vi "SamsGrapher.vi"() -> ()   [LabVIEW 2016]
uses:
  inventory type def.ctl
  subscription type def.ctl
  Communication Global variables.vi
  <vilib>/addons/_JKI.lib/Serialization/JSON/JKI JSON Serialization.lvlib
panel:
  in  "Tab Control":enum32{"Controls", "Graph"}(tab)
  in  "Save Config":bool
  in  "refresh list":bool
  in  "Device selection":i32(listbox)
  in  "Selected parameters":i32[](listbox)
  in  "Available parameters":i32[](listbox)
  in  "Config Button":bool
  out "Data rate (hz)":dbl(knob) scale=0.0..200.0
  in  "Enable graphing":bool=TRUE
  out "Waveform chart":waveform(dbl)[](graph)=[{"t0"=timestamp(3553447770.6895175 s since 1904-01-01), "dt"=1.0, "Y"=[0.0]}, {"t0"=timestamp(3553447770.6895175 s since 1904-01-01), "dt"=1.0, "Y"=[nan]}, {"t0"=timestamp(3553447770.6895175 s since 1904-01-01), "dt"=1.0, "Y"=[nan]}, {"t0"=timestamp(3553447770.6895175 s since 1904-01-01), "dt"=1.0, "Y"=[nan]}, {"t0"=timestamp(3553447770.6895175 s since 1904-01-01), "dt"=1.0, "Y"=[nan]}, {"t0"=timestamp(3553447770.6895175 s since 1904-01-01), "dt"=1.0, "Y"=[nan]}, {"t0"=timestamp(3553447770.6895175 s since 1904-01-01), "dt"=1.0, "Y"=[nan]}, {"t0"=timestamp(3553447770.6895175 s since 1904-01-01), "dt"=1.0, "Y"=[nan]}, {"t0"=timestamp(3553447770.6895175 s since 1904-01-01), "dt"=1.0, "Y"=[nan]}, {"t0"=timestamp(3553447770.6895175 s since 1904-01-01), "dt"=1.0, "Y"=[nan]}, {"t0"=timestamp(3553447770.6895175 s since 1904-01-01), "dt"=1.0, "Y"=[nan]}, {"t0"=timestamp(3553447770.6895175 s since 1904-01-01), "dt"=1.0, "Y"=[nan]}, {"t0"=timestamp(3553447770.6895175 s since 1904-01-01), "dt"=1.0, "Y"=[nan]}, {"t0"=timestamp(3553447770.6895175 s since 1904-01-01), "dt"=1.0, "Y"=[nan]}, {"t0"=timestamp(3553447770.6895175 s since 1904-01-01), "dt"=1.0, "Y"=[nan]}, {"t0"=timestamp(3553447770.6895175 s since 1904-01-01), "dt"=1.0, "Y"=[nan]}]
  out "initialize error":errorcluster
  out "error out":errorcluster
  in  "stop":bool
  # "Parameter Selection"
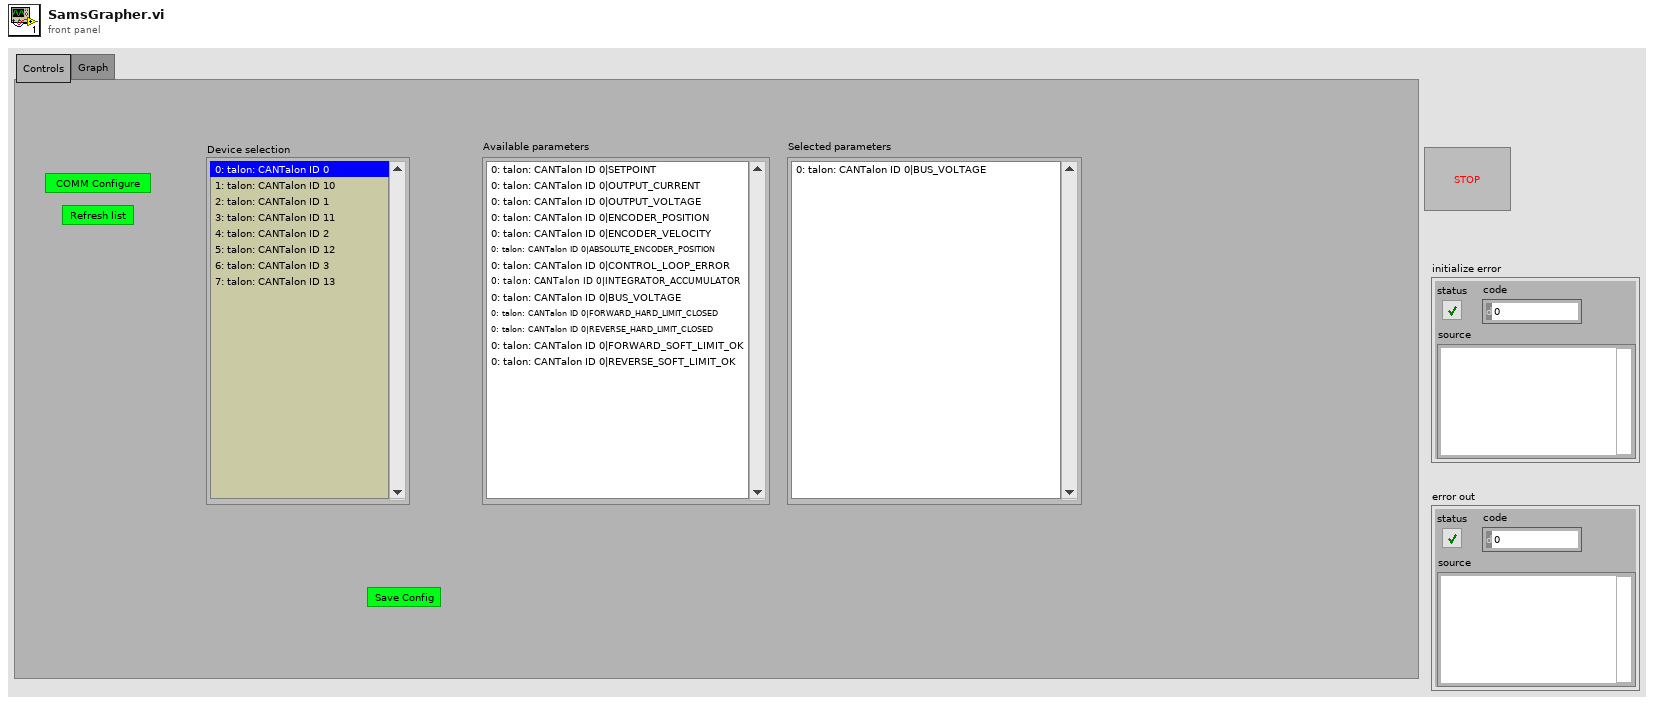
[diagram p1: front panel]
types:
  T1 = typedef "subscription type def.ctl" = cluster{"type":string, "subscription":cluster{"itemId":i32, "measurementId":string}[]}
  T2 = typedef "inventory type def.ctl" = cluster{"items":cluster{"id":u8, "type":string, "description":string}[], "measures":cluster{"deviceType":string, "deviceMeasures":cluster{"id":string, "description":string}[]}[], "type":string}
  T3 = cluster{"type":string, "timestamp":i64, "data":dbl[]}
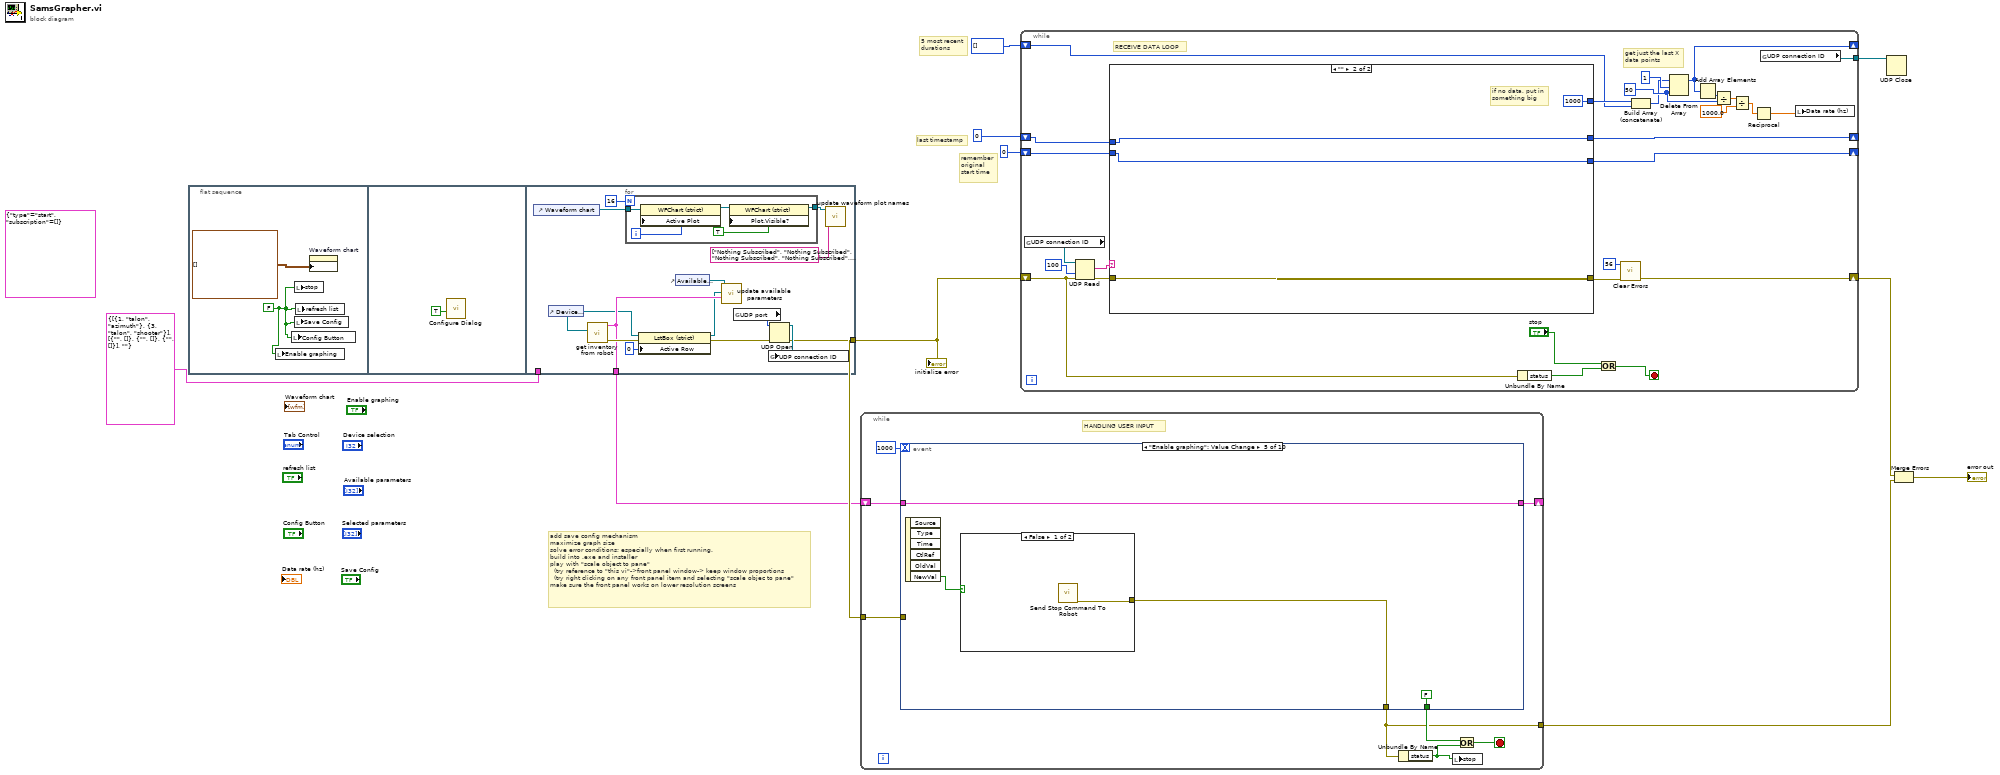
[diagram p0: block diagram]
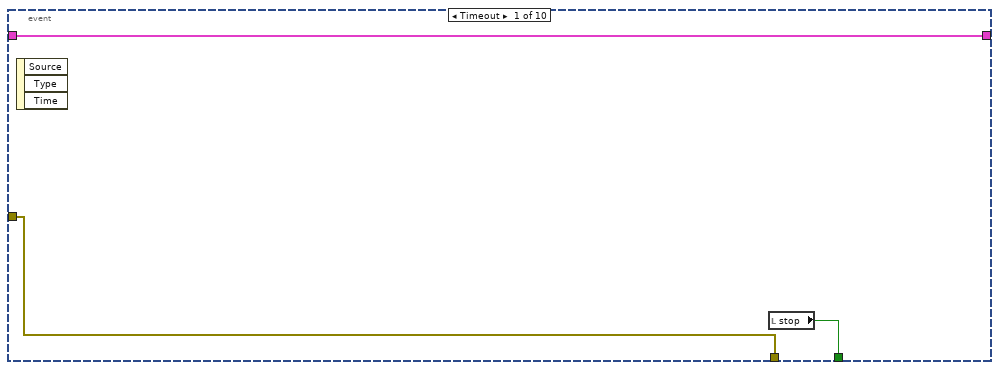
[diagram p2: hidden frame]
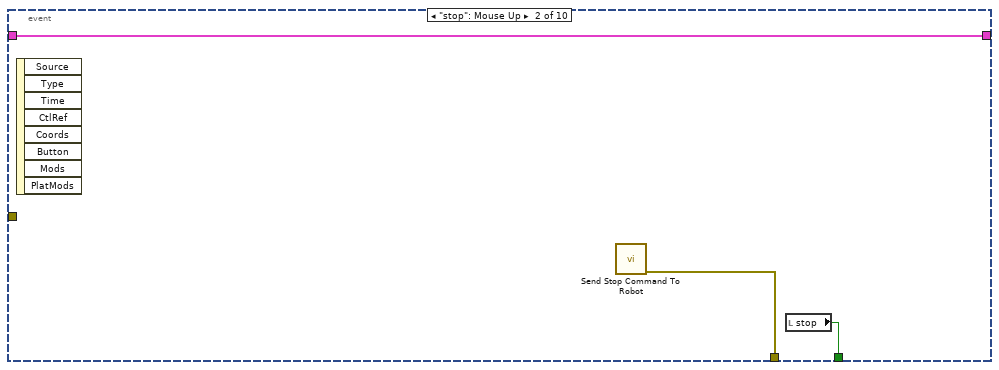
[diagram p3: hidden frame]
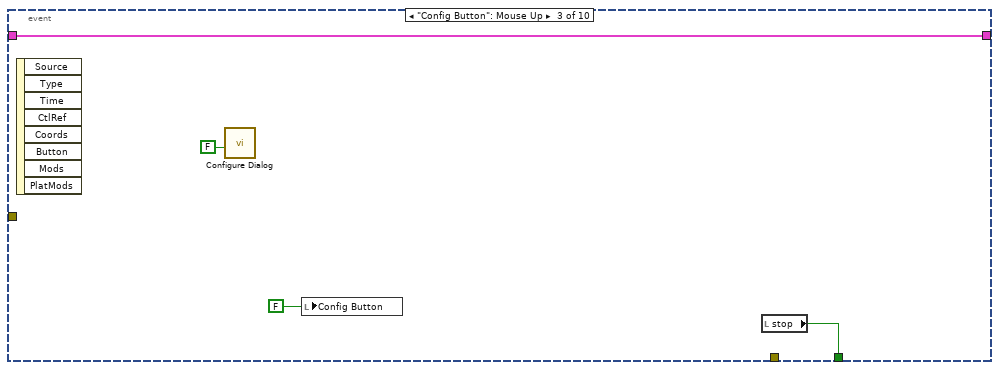
[diagram p4: hidden frame]
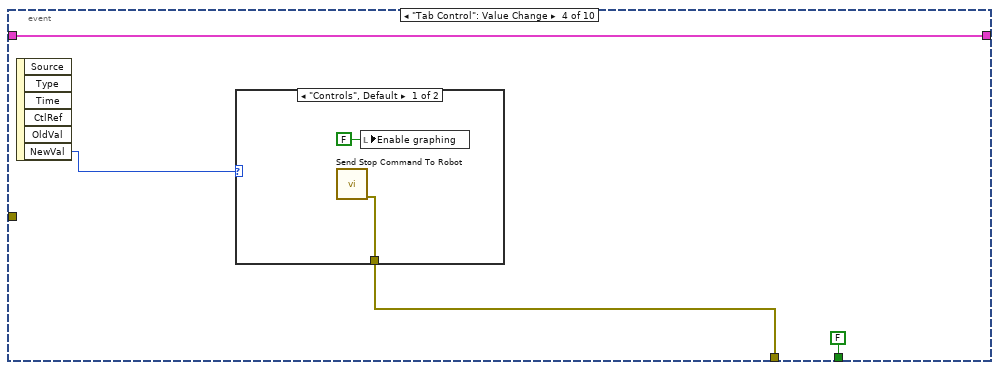
[diagram p5: hidden frame]
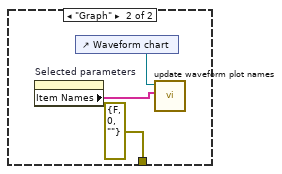
[diagram p6: hidden frame]
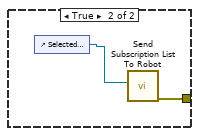
[diagram p7: hidden frame]
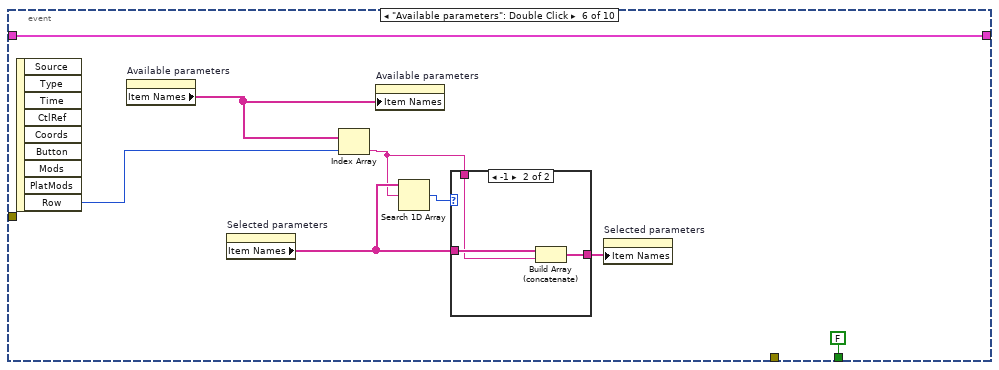
[diagram p8: hidden frame]
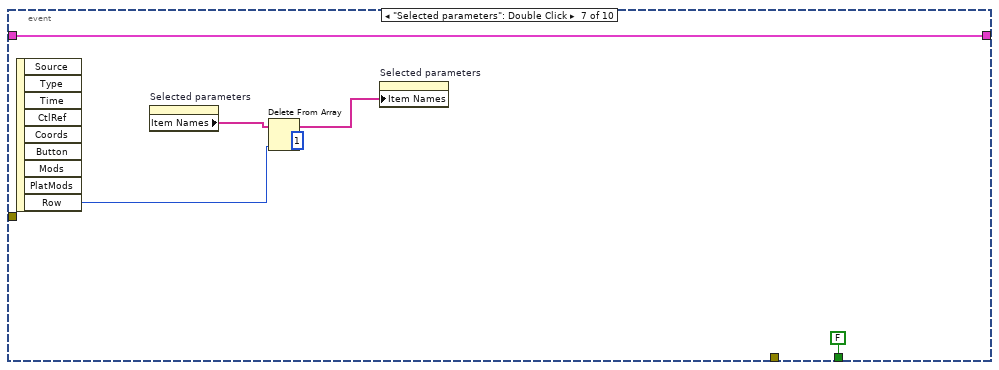
[diagram p10: hidden frame]
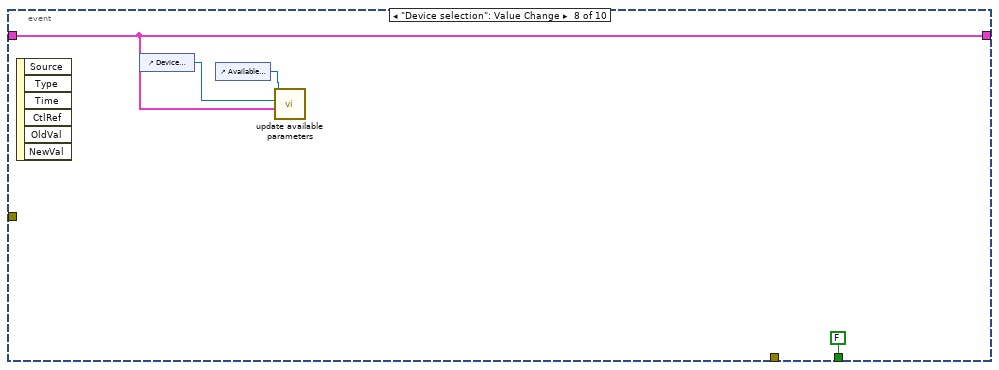
[diagram p11: hidden frame]
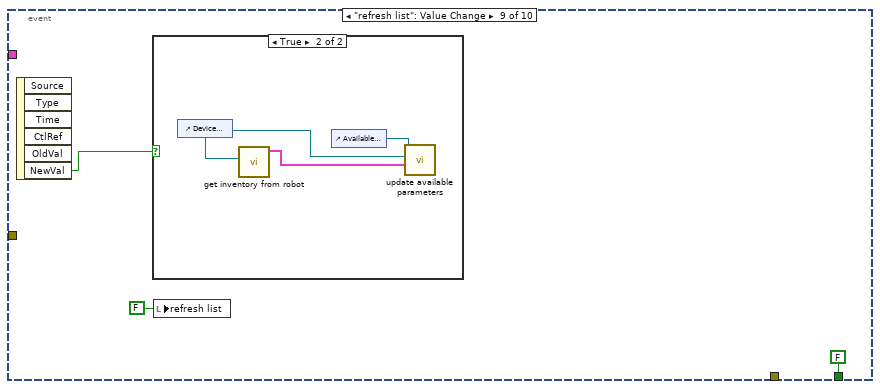
[diagram p12: hidden frame]
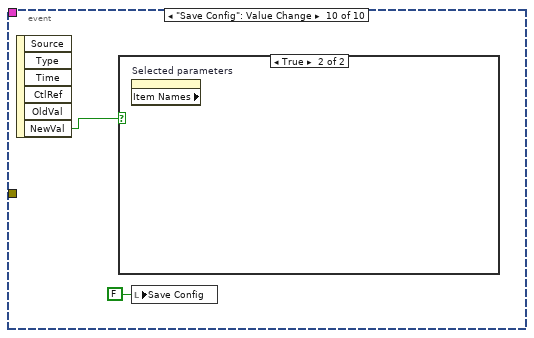
[diagram p14: hidden frame]
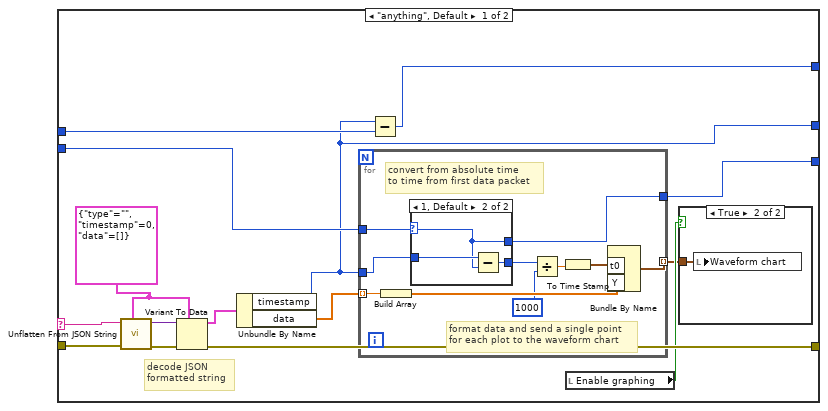
[diagram p16: hidden frame]
diagram:
  (unwired) T1 {"type"="start", "subscription"=[]}
  # "last timestamp"
  # "remember\noriginal\nstart time"
  # "5 most recent\ndurations"
  # "add save config mechanism\nmaximize graph size\nsolve error conditions; especially when first running.\nbuild into .exe and installer\nplay with \"scale object to pane\" \n  (try reference to \"this vi\"->front panel window-> keep window proportions\n  (try right clicking on any front panel item and selecting \"scale objec to pane\"\nmake sure the front panel works on lower resolution screens"
  n1 = flat-sequence {
    tunnel: [w25] -> w7
    tunnel: [w16] -> w6
    tunnel: T2 {"items"=[{"id"=1, "type"="talon", "description"="azimuth"}, {"id"=3, "type"="talon", "description"="shooter"}], "measures"=[{"deviceType"="", "deviceMeasures"=[]}, {"deviceType"="", "deviceMeasures"=[]}, {"deviceType"="", "deviceMeasures"=[]}], "type"=""} -> [_]
    frame #0 {
      w11 = FALSE ("Send")
      n2 = local write "Enable graphing"(w11) -> ()
      n3 = local write "Config Button"(w11) -> ()
      n4 = local write "Save Config"(w11) -> ()
      n5 = local write "stop"(w11) -> ()
      n6 = local write "refresh list"(w11) -> ()
      n7 = property on="Waveform chart" class="WFChart (strict)"("History Data"=waveform(dbl)[][] []) -> ()  [unwired: 2 in, 2 out]
    }
    frame #1 {
      n8 = call "Configure Dialog.vi"("First time?"=TRUE) -> ()  [unwired: 10 in]
    }
    frame #2 {
      n9 = control-ref of="Waveform chart"() -> (w22:refnum<vi>)
      n10 = control-ref of="Device selection"() -> (w14:refnum<vi>)
      n11 = call "get inventory from robot.vi"("Device selection"=w14) -> ("error out"=w19:errorcluster, "Inventory"=w16:T2)  [unwired: 9 in]
      n12 = for {
        N: 16 -> [_]
        tunnel: w22 -> [w32]
        tunnel: [w28] -> w20
        i -> [w30]
        n13 = property class="WFChart (strict)"(reference=w32, "Active Plot"=w30) -> (reference out=w31:refnum<vi>)  [unwired: 1 in, 1 out]
        n14 = property class="WFChart (strict)"(reference=w31, "Plot.Visible?"=TRUE ("Plot.Visible")) -> (reference out=w28:refnum<vi>)  [unwired: 1 in, 1 out]
      }
      n15 = property class="LstBox (strict)"(reference=w14, error in=w19, "Active Row"=0 ("Active Row:Active Row Number")) -> (reference out=w15:refnum<vi>, error out=w18:errorcluster)
      n16 = control-ref of="Available parameters"() -> (w24:refnum<vi>)
      n17 = call "update available parameters.vi"("inventory"=w16, "Device selection"=w15, "Available parameters"=w24) -> ()  [unwired: 9 in]
      n18 = global read "Communication Global variables.vi" "UDP port"() -> (w26:u16)
      n19 = UDP Open(8:w18, 11:w26) -> (port=w27:refnum<k16>, 0:w25:errorcluster)  [unwired: 3 in, 1 out]
      n20 = global write "Communication Global variables.vi" "UDP connection ID"(w27) -> ()
      n21 = call "update waveform plot names.vi"("selected plot names"=string[] ["Nothing Subscribed", "Nothing Subscribed", "Nothing Subscribed", "Nothing Subscribed", "Nothing Subscribed", "Nothing Subscribed", "Nothing Subscribed", "Nothing Subscribed", "Nothing Subscribed", "Nothing Subscribed", "Nothing Subscribed", "Nothing Subscribed", "Nothing Subscribed", "Nothing Subscribed", "Nothing Subscribed", "Nothing Subscribed"], "WaveformChart in"=w20) -> ()  [unwired: 10 in]
    }
  }
  n22 = while {
    tunnel: w7 -> [w38]
    shift-right: [w36] -> _
    shift-left: w6 -> [w37]
    tunnel: [w33] -> w4
    stop <- w40 stop-if-true
    # "HANDLING USER INPUT"
    n23 = event shown="[4] \"Enable graphing\": Value Change" {
      selector: _ -> [_ _ _ _ _ _ _ _ _ _]
      dyn-events: _ -> [_ _ _ _ _ _ _ _ _ _]
      timeout: 1000 -> [_ _ _ _ _ _ _ _ _ _]
      tunnel: [w43 w46 w49 FALSE ("stop") FALSE ("stop") FALSE ("stop") FALSE ("stop") FALSE ("stop") FALSE ("stop") _] -> w35
      tunnel: w38 -> [w41 _ _ _ _ _ _ _ _ _]
      tunnel: w37 -> [w42 w45 w48 w51 w60 w73 w80 w86 _ _]
      tunnel: [w42 w45 w48 w51 w60 w73 w80 w86 _ _] -> w36
      tunnel: [w41 w44 _ w53 w62 _ _ _ _ _] -> w33
      event Timeout {
        n24 = event-data() -> ()  [unwired: 1 in, 3 out]
        n25 = local read "stop"() -> (w43:bool)
      }
      event "stop": Mouse Up {
        n26 = event-data() -> ()  [unwired: 1 in, 8 out]
        n27 = call "Send Stop Command To Robot.vi"() -> ("error out"=w44:errorcluster)  [unwired: 11 in]
        n28 = local read "stop"() -> (w46:bool)
      }
      event "Config Button": Mouse Up {
        n29 = event-data() -> ()  [unwired: 1 in, 8 out]
        n30 = call "Configure Dialog.vi"("First time?"=FALSE) -> ()  [unwired: 10 in]
        n31 = local write "Config Button"(FALSE ("Config Button")) -> ()
        n32 = local read "stop"() -> (w49:bool)
      }
      event "Tab Control": Value Change {
        n33 = event-data() -> ("NewVal"=w54:enum32{"Controls", "Graph"})  [unwired: 1 in, 5 out]
        n34 = case shown="\"Controls\", Default" w54 {
          tunnel: [w56 errorcluster {"status"=FALSE, "code"=0, "source"=""} ("error out")] -> w53
          frame "Controls", Default {
            n35 = call "Send Stop Command To Robot.vi"() -> ("error out"=w56:errorcluster)  [unwired: 11 in]
            n36 = local write "Enable graphing"(FALSE ("Enable graphing")) -> ()
          }
          frame "Graph" {
            n37 = property on="Selected parameters" class="LstBox (strict)"() -> ("Item Names"=w58:string[])  [unwired: 2 in, 2 out]
            n38 = control-ref of="Waveform chart"() -> (w59:refnum<vi>)
            n39 = call "update waveform plot names.vi"("selected plot names"=w58, "WaveformChart in"=w59) -> ()  [unwired: 10 in]
          }
        }
      }
      event "Enable graphing": Value Change {
        n40 = event-data() -> ("NewVal"=w63:bool)  [unwired: 1 in, 5 out]
        n41 = case shown="False" w63 {
          tunnel: [w64 w66] -> w62
          frame False {
            n42 = call "Send Stop Command To Robot.vi"() -> ("error out"=w64:errorcluster)  [unwired: 11 in]
          }
          frame True {
            n43 = control-ref of="Selected parameters"() -> (w65:refnum<vi>)
            n44 = call "Send Subscription List To Robot.vi"("Selected parameters 2"=w65) -> ("error out"=w66:errorcluster)  [unwired: 10 in]
          }
        }
      }
      event "Available parameters": Double Click {
        n45 = event-data() -> ("Row"=w67:i32)  [unwired: 1 in, 8 out]
        n46 = property on="Available parameters" class="LstBox (strict)"() -> ("Item Names"=w68:string[])  [unwired: 2 in, 2 out]
        n47 = property on="Selected parameters" class="LstBox (strict)"() -> ("Item Names"=w71:string[])  [unwired: 2 in, 2 out]
        n48 = Index Array(array=w68, index=w67) -> (element=w69:string)
        n49 = property on="Available parameters" class="LstBox (strict)"("Item Names"=w68) -> ()  [unwired: 2 in, 2 out]
        n50 = Search 1D Array(1D array=w71, element=w69) -> (index of element=w70:i32)  [unwired: 1 in]
        n51 = case shown="-1" w70 {
          tunnel: [w75 w78] -> w74
          tunnel: w71 -> [w75 w77]
          tunnel: w69 -> [_ w76]
          frame 0, Default {
          }
          frame -1 {
            n52 = Build Array (concatenate)(w77, w76) -> (w78:string[])
          }
        }
        n53 = property on="Selected parameters" class="LstBox (strict)"("Item Names"=w74) -> ()  [unwired: 2 in, 2 out]
      }
      event "Selected parameters": Double Click {
        n54 = event-data() -> ("Row"=w82:i32)  [unwired: 1 in, 8 out]
        n55 = property on="Selected parameters" class="LstBox (strict)"() -> ("Item Names"=w84:string[])  [unwired: 2 in, 2 out]
        n56 = Delete From Array(array=w84, length=1, index=w82) -> (array with subset deleted=w81:string[])  [unwired: 1 out]
        n57 = property on="Selected parameters" class="LstBox (strict)"("Item Names"=w81) -> ()  [unwired: 2 in, 2 out]
      }
      event "Device selection": Value Change {
        n58 = event-data() -> ()  [unwired: 1 in, 6 out]
        n59 = control-ref of="Device selection"() -> (w85:refnum<vi>)
        n60 = control-ref of="Available parameters"() -> (w88:refnum<vi>)
        n61 = call "update available parameters.vi"("inventory"=w86, "Device selection"=w85, "Available parameters"=w88) -> ()  [unwired: 9 in]
      }
      event "refresh list": Value Change {
        n62 = event-data() -> ("NewVal"=w91:bool)  [unwired: 1 in, 5 out]
        n63 = case shown="True" w91 {
          frame False {
          }
          frame True {
            n64 = control-ref of="Device selection"() -> (w93:refnum<vi>)
            n65 = call "get inventory from robot.vi"("Device selection"=w93) -> ("Inventory"=w92:T2)  [unwired: 9 in, 1 out]
            n66 = control-ref of="Available parameters"() -> (w94:refnum<vi>)
            n67 = call "update available parameters.vi"("inventory"=w92, "Device selection"=w93, "Available parameters"=w94) -> ()  [unwired: 9 in]
          }
        }
        n68 = local write "refresh list"(FALSE ("refresh list")) -> ()
      }
      event "Save Config": Value Change {
        n69 = event-data() -> ("NewVal"=w96:bool)  [unwired: 1 in, 5 out]
        n70 = case shown="True" w96 {
          frame False {
          }
          frame True {
            n71 = property on="Selected parameters" class="LstBox (strict)" props=["Item Names"]() -> ()  [unwired: 2 in, 3 out]
          }
        }
        n72 = local write "Save Config"(FALSE ("Save Config")) -> ()
      }
    }
    n73 = Unbundle By Name(w33) -> ("status"=w34:bool)
    n74 = local write "stop"(w34) -> ()
    n75 = Or(x=w35, y=w34) -> (x .or. y?=w40:bool)
  }
  n76 = while {
    shift-right: [w120] -> w10
    shift-left: w7 -> [w118]
    tunnel: [w112] -> w8
    shift-right: [w110] -> _
    shift-left: i64 0 ("timestamp") -> [w111]
    shift-right: [w97] -> _
    shift-left: i64[] [] -> [w98]
    shift-right: [w108] -> _
    shift-left: i64 0 ("timestamp") -> [w109]
    stop <- w121 stop-if-true
    w103 = 50 ("index")
    # "get just the last X\ndata points"
    # "RECEIVE DATA LOOP"
    n77 = global read "Communication Global variables.vi" "UDP connection ID"() -> (w113:refnum<k16>)
    n78 = UDP Read(connection ID=w113, timeout ms (25000)=100, 8:w118) -> (data out=w116:string, error out=w117:errorcluster)  [unwired: 1 in, 3 out]
    n79 = case shown="\"\"" w116 {
      selector: w116 -> [w137 _]
      tunnel: w117 -> [w138 w158]
      tunnel: [w134 w158] -> w114
      tunnel: w111 -> [w128 w157]
      tunnel: [w127 w157] -> w110
      tunnel: w109 -> [w126 w156]
      tunnel: [w125 w156] -> w108
      tunnel: [w124 i64 1000] -> w99
      frame "anything", Default {
        w131 = T3 {"type"="", "timestamp"=0, "data"=[]}
        # "decode JSON\nformatted string"
        n80 = call <vilib>:"Unflatten From JSON String.vi"("Type and Defaults"=w131, "error in (no error)"=w138, "JSON String"=w137) -> ("error out"=w136:errorcluster, "Variant"=w135:variant)  [unwired: 7 in]
        n81 = Variant To Data(error in=w136, type=w131, Variant=w135) -> (data=w133:T3, error out=w134:errorcluster)
        n82 = Unbundle By Name(w133) -> ("timestamp"=w125:i64, "data"=w132:dbl[])
        n83 = for {
          tunnel: w125 -> [w145]
          tunnel: [w148] -> w129 mode=indexing
          tunnel: w132 -> [w147] mode=indexing
          tunnel: w128 -> [w144]
          tunnel: [w143] -> w127
          # "convert from absolute time\nto time from first data packet"
          # "format data and send a single point\nfor each plot to the waveform chart"
          n84 = Build Array(w147) -> (w149:dbl[])
          n85 = case shown="1, Default" w144 {
            selector: w144 -> [w151 w152]
            tunnel: [w151 w154] -> w140
            tunnel: w145 -> [w150 w153]
            tunnel: [w150 w152] -> w143
            frame 0 {
            }
            frame 1, Default {
              n86 = Subtract(x=w153, y=w152) -> (x-y=w154:i64)
            }
          }
          n87 = Divide(x=w140, y=i64 1000) -> (x/y=w142:dbl)
          n88 = To Time Stamp(1:w142) -> (0:w146:timestamp)
          n89 = Bundle By Name("t0"=w146, "Y"=w149) -> (w148:waveform(dbl))  [unwired: 1 in]
        }
        n90 = Subtract(x=w125, y=w126) -> (x-y=w124:i64)
        n91 = local read "Enable graphing"() -> (w130:bool)
        n92 = case shown="True" w130 {
          tunnel: w129 -> [_ w139]
          frame False {
          }
          frame True {
            n93 = local write "Waveform chart"(w139) -> ()
          }
        }
      }
      frame "" {
        # "if no data, put in\nsomething big"
      }
    }
    n94 = Unbundle By Name(w118) -> ("status"=w123:bool)
    n95 = Or(x="stop", y=w123) -> (x .or. y?=w121:bool)
    n96 = call <vilib>:"Clear Errors.vi"("error in (no error)"=w114, "specific error code to clear (0: all)"=56) -> ("error out"=w120:errorcluster)  [unwired: 4 in, 1 out]
    n97 = Build Array (concatenate)(w99, w98) -> (w100:i64[])
    n98 = Delete From Array(array=w100, length=1, index=w103) -> (array with subset deleted=w97:i64[])  [unwired: 1 out]
    n99 = Add Array Elements(numeric array=w97) -> (sum=w102:i64)
    n100 = Divide(x=w102, y=w103) -> (x/y=w104:dbl)
    n101 = Divide(x=w104, y=1000.0) -> (x/y=w106:dbl)
    n102 = Reciprocal(x=w106) -> (1/x=w107:dbl)
    n103 = global read "Communication Global variables.vi" "UDP connection ID"() -> (w112:refnum<k16>)
    n104 = local write "Data rate (hz)"(w107) -> ()
  }
  n105 = UDP Close(connection ID=w8) -> ()  [unwired: 1 in, 2 out]
  n106 = Merge Errors(w10, w4) -> (→"error out":errorcluster)
  "initialize error" <- w7
